vi "Configure Spectrum Emission Mask (Sweep Trace Setup).vi"(0 "VISA resource name":refnum<visa-resource-name>, 1 "SEM Point (12:10001)":i32(ring)=12 items=["11", "21", "41", "51", "101", "201", "251", "401", "501", "1001", "2001", "5001", "10001"], 5 "SEM Auto Sweep Time (1:On)":i32(ring)=1 items=["Off", "On"], 7 "SEM Sweep Speed Select (0:Normal)":i32(ring) items=["Normal", "Fast"], 9 "SEM Sweep Time (0.04s)":dbl=0.04 min=0.001 max=1000.0, 11 "error in (no error)":errorcluster, 12 "SEM Detection Mode (0:Pos and Neg Peaks)":i32(ring) items=["Pos and Neg Peaks", "Positive Peaks", "Negative Peaks", "Sampling", "RMS"]) -> (4 "VISA resource name out":refnum<visa-resource-name>, 15 "error out":errorcluster)   [LabVIEW 2020, in "Anritsu Signal Analyzer Series.lvlib"]
doc: "Configures the sweep and trace parameter for reference of SEM measurement settings of the spectrum analyzer."
uses:
  Anritsu Signal Analyzer Series.lvlib
panel:
  # "s"
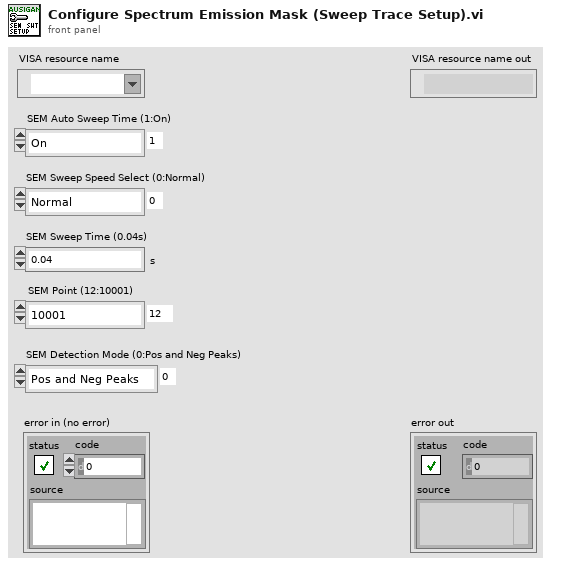
[diagram p1: front panel]
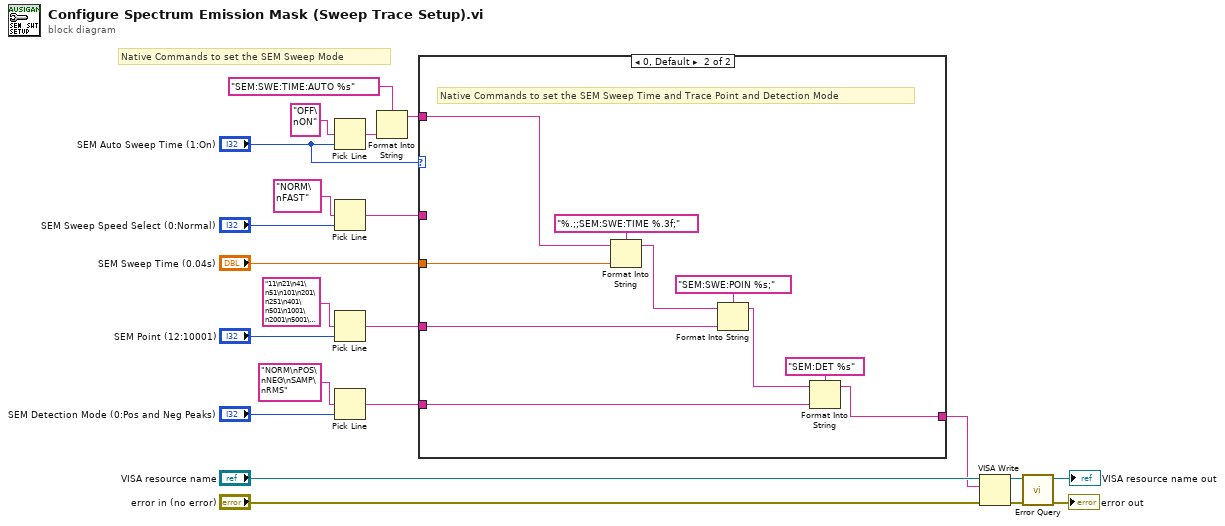
[diagram p0: block diagram]
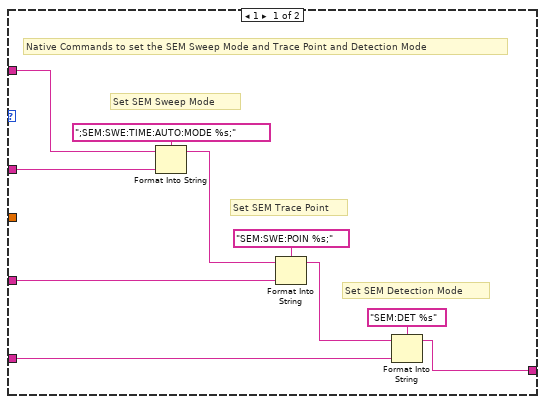
[diagram p2: hidden frame]
diagram:
  # "Native Commands to set the SEM Sweep Mode"
  n1 = Pick Line(multi-line string="OFF\nON" ("複数行文字列"), line index="SEM Auto Sweep Time (1:On)") -> (output string=w9:string)  [unwired: 1 in]
  n2 = Pick Line(multi-line string="NORM\nFAST" ("複数行文字列"), line index="SEM Sweep Speed Select (0:Normal)") -> (output string=w7:string)  [unwired: 1 in]
  n3 = Pick Line(multi-line string="11\n21\n41\n51\n101\n201\n251\n401\n501\n1001\n2001\n5001\n10001" ("複数行文字列"), line index="SEM Point (12:10001)") -> (output string=w4:string)  [unwired: 1 in]
  n4 = Pick Line(multi-line string="NORM\nPOS\nNEG\nSAMP\nRMS" ("複数行文字列"), line index="SEM Detection Mode (0:Pos and Neg Peaks)") -> (output string=w5:string)  [unwired: 1 in]
  n5 = Format Into String(format string="SEM:SWE:TIME:AUTO %s" ("_CommandSet"), w9) -> (resulting string=w11:string)  [unwired: 2 in, 1 out]
  n6 = case shown="0, Default" "SEM Auto Sweep Time (1:On)" {
    tunnel: w7 -> [w32 _]
    tunnel: w11 -> [w31 w35]
    tunnel: "SEM Sweep Time (0.04s)" -> [_ w34]
    tunnel: w5 -> [w28 w39]
    tunnel: [w25 w36] -> w13
    tunnel: w4 -> [w23 w33]
    frame 1 {
      # "Native Commands to set the SEM Sweep Mode and Trace Point and Detection Mode"
      # "Set SEM Detection Mode"
      # "Set SEM Trace Point"
      # "Set SEM Sweep Mode"
      n7 = Format Into String(format string=";SEM:SWE:TIME:AUTO:MODE %s;" ("_CommandSet"), initial string=w31, w32) -> (resulting string=w24:string)  [unwired: 1 in, 1 out]
      n8 = Format Into String(format string="SEM:SWE:POIN %s;" ("Format String"), initial string=w24, w23) -> (resulting string=w27:string)  [unwired: 1 in, 1 out]
      n9 = Format Into String(format string="SEM:DET %s" ("_CommandSet"), initial string=w27, w28) -> (resulting string=w25:string)  [unwired: 1 in, 1 out]
    }
    frame 0, Default {
      # "Native Commands to set the SEM Sweep Time and Trace Point and Detection Mode"
      n10 = Format Into String(format string="%.;;SEM:SWE:TIME %.3f;" ("Format String"), initial string=w35, w34) -> (resulting string=w40:string)  [unwired: 1 in, 1 out]
      n11 = Format Into String(format string="SEM:SWE:POIN %s;" ("Format String"), initial string=w40, w33) -> (resulting string=w38:string)  [unwired: 1 in, 1 out]
      n12 = Format Into String(format string="SEM:DET %s" ("_CommandSet"), initial string=w38, w39) -> (resulting string=w36:string)  [unwired: 1 in, 1 out]
    }
  }
  n13 = VISA Write(VISA resource name="VISA resource name", write buffer=w13, error in (no error)="error in (no error)") -> (VISA resource name out=w14:refnum<visa-resource-name>, error out=w15:errorcluster)  [unwired: 1 out]
  n14 = call "Error Query.vi"("error in (no error)"=w15, "VISA resource name"=w14) -> ("error out"=→"error out":errorcluster, "VISA resource name out"=→"VISA resource name out":refnum<visa-resource-name>)  [unwired: 6 in, 2 out]
